vi "Untitled 2 (SubVI).vi"(11 "?":T1) -> (3 "appended array":u32[](array[numeric]))   [LabVIEW 2015, in "PolyVIEW.lvclass"]
uses:
  PolyVIEW.lvclass
  Memory.ctl
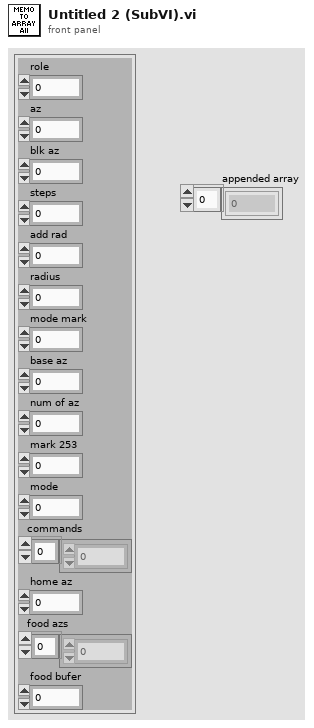
[diagram p1: front panel]
types:
  T1 = typedef "PolyVIEW.lvclass/Memory.ctl" = cluster{"role":i32, "az":i32, "blk az":i32, "steps":u32, "add rad":i32, "radius":dbl, "mode mark":u32, "base az":dbl, "num of az":u32, "mark 253":u32, "mode":u32, "commands":i32[], "home az":dbl, "food azs":dbl[], "food bufer":dbl}
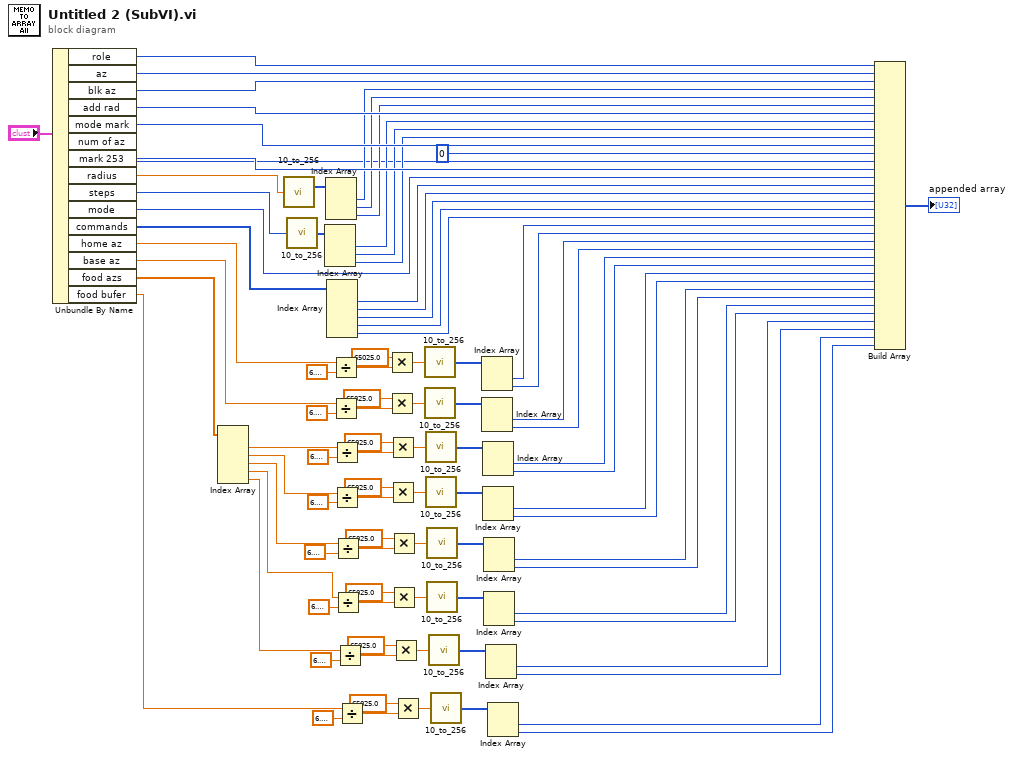
[diagram p0: block diagram]
diagram:
  n1 = Unbundle By Name("?") -> ("role"=w78:i32, "az"=w79:i32, "blk az"=w80:i32, "add rad"=w85:i32, "mode mark"=w90:u32, "num of az"=w68:u32, "mark 253"=w91:u32, "radius"=w76:dbl, "steps"=w67:u32, "mode"=w75:u32, "commands"=w74:i32[], "home az"=w65:dbl, "base az"=w50:dbl, "food azs"=w49:dbl[], "food bufer"=w9:dbl)
  n2 = Index Array(array=w49) -> (element #1=w44:dbl, element #2=w39:dbl, element #3=w34:dbl, element #4=w29:dbl, element #5=w24:dbl)  [unwired: 5 in]
  n3 = call "10_to_256.vi"("Decimal"=w76) -> ("256"=w81:u8[])
  n4 = call "10_to_256.vi"("Decimal"=w67) -> ("256"=w86:u8[])
  n5 = Index Array(array=w86) -> (element #1=w87:u8, element #2=w88:u8, element #3=w89:u8)  [unwired: 3 in]
  n6 = Index Array(array=w81) -> (element #1=w82:u8, element #2=w83:u8, element #3=w84:u8)  [unwired: 3 in]
  n7 = Index Array(array=w74) -> (element #1=w73:i32, element #2=w72:i32, element #3=w71:i32, element #4=w70:i32, element #5=w69:i32)  [unwired: 5 in]
  n8 = Divide(x=w65, y=6.283185307179586) -> (x/y=w66:dbl)
  n9 = Divide(x=w50, y=6.283185307179586) -> (x/y=w58:dbl)
  n10 = Divide(x=w44, y=6.283185307179586) -> (x/y=w48:dbl)
  n11 = Divide(x=w39, y=6.283185307179586) -> (x/y=w43:dbl)
  n12 = Divide(x=w34, y=6.283185307179586) -> (x/y=w38:dbl)
  n13 = Divide(x=w29, y=6.283185307179586) -> (x/y=w33:dbl)
  n14 = Divide(x=w24, y=6.283185307179586) -> (x/y=w28:dbl)
  n15 = Divide(x=w9, y=6.283185307179586) -> (x/y=w13:dbl)
  n16 = Multiply(x=65025.0 ("y"), y=w66) -> (x*y=w64:dbl)
  n17 = Multiply(x=65025.0 ("y"), y=w58) -> (x*y=w57:dbl)
  n18 = Multiply(x=65025.0 ("y"), y=w48) -> (x*y=w47:dbl)
  n19 = Multiply(x=65025.0 ("y"), y=w43) -> (x*y=w42:dbl)
  n20 = Multiply(x=65025.0 ("y"), y=w38) -> (x*y=w37:dbl)
  n21 = Multiply(x=65025.0 ("y"), y=w33) -> (x*y=w32:dbl)
  n22 = Multiply(x=65025.0 ("y"), y=w28) -> (x*y=w27:dbl)
  n23 = Multiply(x=65025.0 ("y"), y=w13) -> (x*y=w12:dbl)
  n24 = call "10_to_256.vi"("Decimal"=w64) -> ("256"=w61:u8[])
  n25 = call "10_to_256.vi"("Decimal"=w57) -> ("256"=w54:u8[])
  n26 = call "10_to_256.vi"("Decimal"=w47) -> ("256"=w45:u8[])
  n27 = call "10_to_256.vi"("Decimal"=w42) -> ("256"=w40:u8[])
  n28 = call "10_to_256.vi"("Decimal"=w37) -> ("256"=w35:u8[])
  n29 = call "10_to_256.vi"("Decimal"=w32) -> ("256"=w30:u8[])
  n30 = call "10_to_256.vi"("Decimal"=w27) -> ("256"=w25:u8[])
  n31 = call "10_to_256.vi"("Decimal"=w12) -> ("256"=w10:u8[])
  n32 = Index Array(array=w61) -> (element #1=w60:u8, element #2=w59:u8)  [unwired: 2 in]
  n33 = Index Array(array=w54) -> (element #1=w53:u8, element #2=w52:u8)  [unwired: 2 in]
  n34 = Index Array(array=w45) -> (element #1=w23:u8, element #2=w22:u8)  [unwired: 2 in]
  n35 = Index Array(array=w40) -> (element #1=w21:u8, element #2=w20:u8)  [unwired: 2 in]
  n36 = Index Array(array=w35) -> (element #1=w19:u8, element #2=w18:u8)  [unwired: 2 in]
  n37 = Index Array(array=w30) -> (element #1=w17:u8, element #2=w16:u8)  [unwired: 2 in]
  n38 = Index Array(array=w25) -> (element #1=w15:u8, element #2=w14:u8)  [unwired: 2 in]
  n39 = Index Array(array=w10) -> (element #1=w8:u8, element #2=w7:u8)  [unwired: 2 in]
  n40 = Build Array(w78, w79, w80, w82, w83, w84, w85, w87, w88, w89, w90, u32 0 ("element"), w68, w91, w75, w73, w72, w71, w70, w69, w60, w59, w53, w52, w23, w22, w21, w20, w19, w18, w17, w16, w15, w14, w8, w7) -> (→"appended array":u32[])
